vi "Read Msg Attributes.vi"(11 "Actor in":refnum<class "Actor.lvclass">) -> (2 "Msg Attributes":refnum<data-value>)   [LabVIEW 2020, in "jettl.lvlib" / "Actor.lvclass"]
uses:
  Actor.lvclass
  Relation.ctl
  jettl.lvlib
  Teller.ctl
  Msg Attributes.ctl
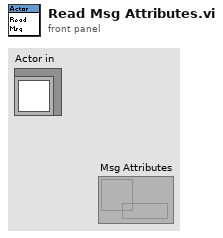
[diagram p1: front panel]
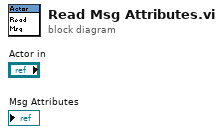
[diagram p0: block diagram]
diagram:
